vi "系统全局变量.vi"() -> ()   [LabVIEW 2014]
panel:
  out "实验上位机路径":path
  out "系统根路径":path
  out "在线时间":string
  out "实验名":string
  out "学号":string
  out "姓名":string
  # "用户和实验信息"
  # "路径"
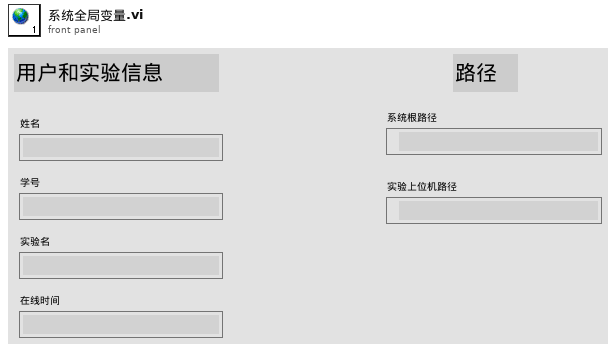
[diagram p1: front panel]
diagram:
